vi "Teleop.vi"(10 "Match Info":T1={"Autonomous Elapsed Seconds"=0.0, "TeleOp Elapsed Seconds"=0.0, "Disabled Elapsed Seconds"=0.0, "Visited Autonomous"=FALSE, "Visited TeleOp"=FALSE, "Visited Disabled"=FALSE, "Autonomous Settings"={"Autonomous Style"=enum."Independent", "VI Refnum"=refnum}}, 11 "Call Context":T2) -> ()   [LabVIEW 2014]
doc: "This VI is called for each TeleOp packet received from the DS where the robot is not disabled. It is often used to read from the joysticks and update I/O or to update setpoints for timed control loops. It should complete and return within 20 milliseconds or it may miss DS packets."
uses:
  <vilib>/Rock Robotics/WPI/DriverStation/WPI_DriverStationDerivedRobotMode.ctl
  <vilib>/Rock Robotics/WPI/DriverStation/WPI_DriverStationMatch Info.ctl
  <vilib>/Rock Robotics/Network Tables/SD Read Boolean.vi
  <vilib>/Rock Robotics/Network Tables/SD Read Number.vi
panel:
  out "Seconds Left in Match":dbl
  out "Sample Slider 0":dbl(slide) scale=0.0..5.0
  out "Sample Boolean 1":bool
  out "Sample Boolean 0":bool
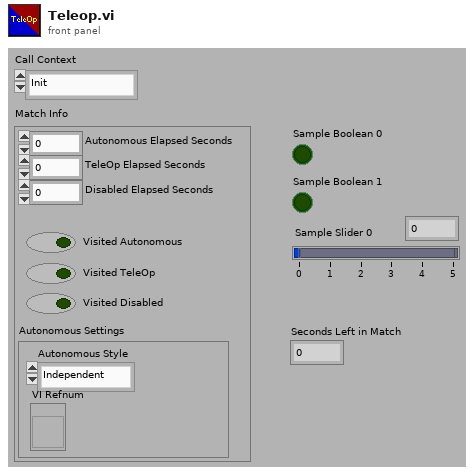
[diagram p1: front panel]
types:
  T1 = typedef "WPI_DriverStationMatch Info.ctl" = cluster{"Autonomous Elapsed Seconds":dbl, "TeleOp Elapsed Seconds":dbl, "Disabled Elapsed Seconds":dbl, "Visited Autonomous":bool, "Visited TeleOp":bool, "Visited Disabled":bool, "Autonomous Settings":cluster{"Autonomous Style":enum16{"Iterative", "Independent"}, "VI Refnum":refnum<vi>}}
  T2 = typedef "WPI_DriverStationDerivedRobotMode.ctl" = enum16{"Init", "Execute", "Stop"}
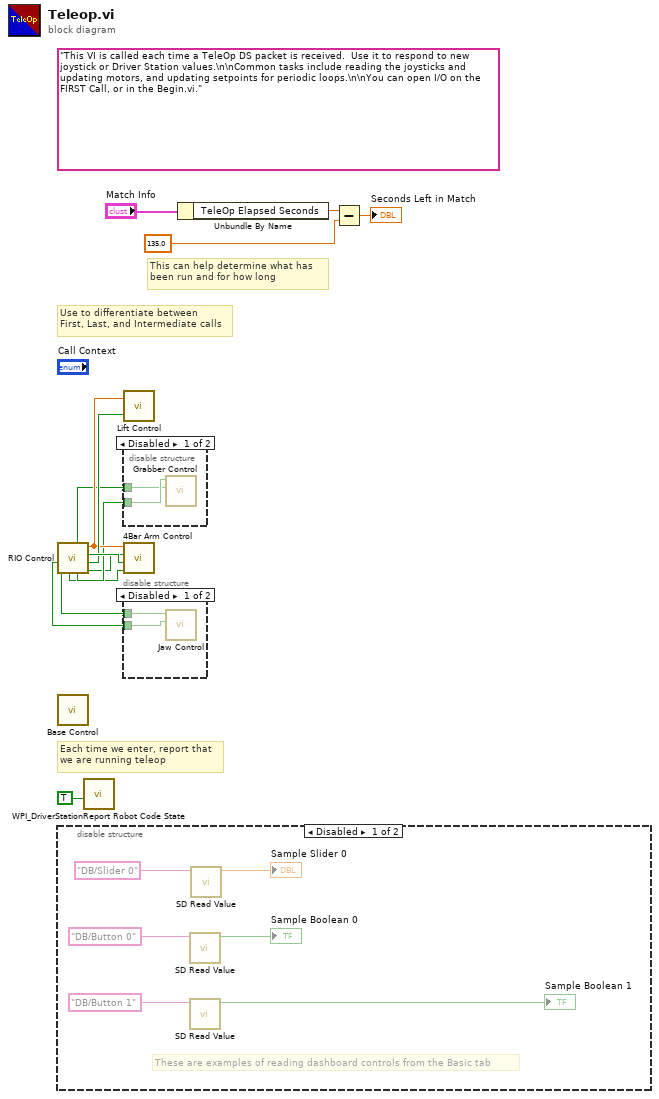
[diagram p0: block diagram]
diagram:
  (unwired) "This VI is called each time a TeleOp DS packet is received.  Use it to respond to new joystick or Driver Station values.\n\nCommon tasks include reading the joysticks and updating motors, and updating setpoints for periodic loops.\n\nYou can open I/O on the FIRST Call, or in the Begin.vi."
  # "Each time we enter, report that\nwe are running teleop"
  # "Use to differentiate between\nFirst, Last, and Intermediate calls"
  # "This can help determine what has\nbeen run and for how long"
  n1 = call "RIO Control.vi"() -> ("Disable Sensors"=w5:bool, "Lift Control"=w11:bool, "4Bar Control"=w12:bool, "Joystick Value"=w10:dbl, "Grabber Inhale"=w7:bool, "Grabber Exhale"=w6:bool, "B8 - Enable Arm Setpoint"=w1:bool, "Jaw Open"=w9:bool, "Jaw Close"=w8:bool)  [unwired: 3 in]
  n2 = call "Base Control.vi"() -> ()  [unwired: 1 in, 2 out]
  n3 = disable-structure shown="Disabled" {
    frame Disabled {
      # "These are examples of reading dashboard controls from the Basic tab"
      n4 = call-poly <vilib>:"SD Read Value.vi"("Name"="DB/Button 0" ("refnum name")) -> ("Boolean"=→"Sample Boolean 0":bool)  [unwired: 8 in, 2 out]
      n5 = call-poly <vilib>:"SD Read Value.vi"("Name"="DB/Button 1" ("refnum name")) -> ("Boolean"=→"Sample Boolean 1":bool)  [unwired: 8 in, 2 out]
      n6 = call-poly <vilib>:"SD Read Value.vi"("Name"="DB/Slider 0" ("refnum name")) -> ("Numeric"=→"Sample Slider 0":dbl)  [unwired: 8 in, 2 out]
    }
    frame Enabled {
    }
  }
  n7 = call <vilib>:"WPI_DriverStationReport Robot Code State.vi"("TeleOp"=TRUE ("Autonomous")) -> ()  [unwired: 10 in, 1 out]
  n8 = call "Lift Control.vi"("Joystick Input"=w10, "Lift Control"=w11) -> ()  [unwired: 4 in]
  n9 = disable-structure shown="Disabled" {
    disable-tunnel: w7 -> [w22 _]
    disable-tunnel: w6 -> [w21 _]
    frame Disabled {
      n10 = call "Grabber Control.vi"("Arm Motor Exhale Tote"=w21, "Arm Motor Inhale Tote"=w22) -> ()  [unwired: 8 in]
    }
    frame Enabled {
    }
  }
  n11 = call "4Bar Arm Control.vi"("Enable Setup"=w1, "4Bar Button"=w12, "Disable Sensor"=w5, "Joystick Input"=w10) -> ()  [unwired: 8 in]
  n12 = disable-structure shown="Disabled" {
    disable-tunnel: w9 -> [w24 _]
    disable-tunnel: w8 -> [w23 _]
    frame Disabled {
      n13 = call "Jaw Control.vi"("Jaw Close"=w23, "Jaw Open"=w24) -> ()  [unwired: 8 in]
    }
    frame Enabled {
    }
  }
  n14 = Unbundle By Name("Match Info") -> ("TeleOp Elapsed Seconds"=w4:dbl)
  n15 = Subtract(x=w4, y=135.0) -> (x-y=→"Seconds Left in Match":dbl)
